vi "GenerateCode.vi"(0 "XRef":T17, 1 "Terms":T14, 2 "Diagram":T13, 3 "State In":T1) -> (14 "Generated Code?":T9, 15 "Reply":T12, 16 "Fatal Error Out":T11, 17 "State Out":T1)   [LabVIEW 2021, in "myRIO AO N Samples Open.xnode"]
uses:
  <vilib>/myRIO/Instrument Drivers/Onboard IO/AO Block/vis/myRIO AO N Samples Open.xnode
  <vilib>/XNodeSupport/XNodeXNodeRef.ctl
  <vilib>/XNodeSupport/XNodeTermIDPairs.ctl
  <vilib>/XNodeSupport/XNodeTermIDPair.ctl
  <vilib>/XNodeSupport/XNodeTermRef.ctl
  <vilib>/XNodeSupport/XNodeString.ctl
  <vilib>/XNodeSupport/XNodeTopLevelDiagramRef.ctl
  <vilib>/myRIO/Instrument Drivers/Onboard IO/AO Block/vis/State.ctl
  <vilib>/myRIO/Common/Instrument Driver Framework/Utilities/typedefs/myRIOXPeripheral.ctl
  <vilib>/XNodeSupport/XNodeTerm4Array.ctl
  <vilib>/XNodeSupport/XNodeTerm4.ctl
  <vilib>/XNodeSupport/XNodeVariant.ctl
  <vilib>/XNodeSupport/XNodeRect32.ctl
  <vilib>/XNodeSupport/XNodeInt.ctl
  <vilib>/XNodeSupport/XNodeBool.ctl
  <vilib>/XNodeSupport/XNodeTermDirection.ctl
  <vilib>/XNodeSupport/XNodeStringArray.ctl
  <vilib>/XNodeSupport/XNodeErrorCluster.ctl
  <vilib>/userdefined/High Color/nirio_resource_hc.ctl
  <vilib>/XNodeSupport/NI_XNodeSupport.lvlib
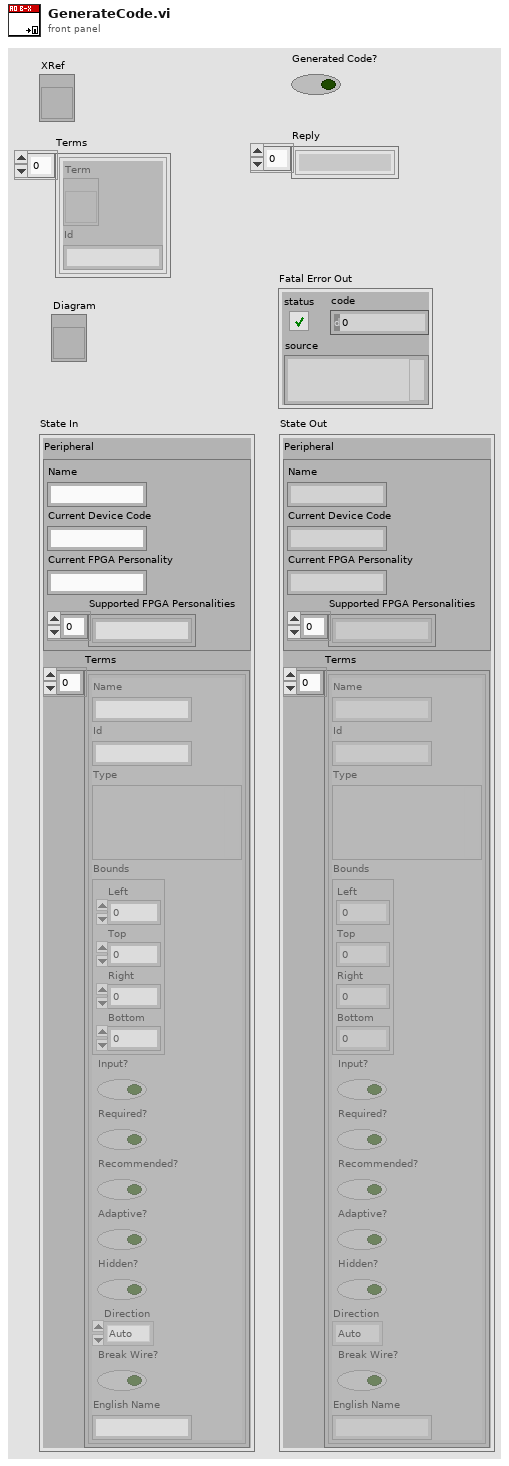
[diagram p1: front panel]
types:
  T1 = typedef "myRIO AO N Samples Open.xnode/State.ctl" = cluster{"Peripheral":T2, "Terms":T3}
  T2 = typedef "myRIOXPeripheral.ctl" = cluster{"Name":string, "Current Device Code":string, "Current FPGA Personality":string, "Supported FPGA Personalities":string[]}
  T3 = typedef "NI_XNodeSupport.lvlib/XNodeTerm4Array.ctl" = T4[]
  T4 = typedef "NI_XNodeSupport.lvlib/XNodeTerm4.ctl" = cluster{"Name":T5, "Id":T5, "Type":T6, "Bounds":T7, "Input?":T9, "Required?":T9, "Recommended?":T9, "Adaptive?":T9, "Hidden?":T9, "Direction":T10, "Break Wire?":T9, "English Name":T5}
  T5 = typedef "NI_XNodeSupport.lvlib/XNodeString.ctl" = string
  T6 = typedef "NI_XNodeSupport.lvlib/XNodeVariant.ctl" = variant
  T7 = typedef "NI_XNodeSupport.lvlib/XNodeRect32.ctl" = cluster{"Left":T8, "Top":T8, "Right":T8, "Bottom":T8}
  T8 = typedef "NI_XNodeSupport.lvlib/XNodeInt.ctl" = i32
  T9 = typedef "NI_XNodeSupport.lvlib/XNodeBool.ctl" = bool
  T10 = typedef "NI_XNodeSupport.lvlib/XNodeTermDirection.ctl" = enum32{"Auto", "Up", "Down", "Left", "Right", "Center"}
  T11 = typedef "NI_XNodeSupport.lvlib/XNodeErrorCluster.ctl" = errorcluster
  T12 = typedef "NI_XNodeSupport.lvlib/XNodeStringArray.ctl" = T5[]
  T13 = typedef "NI_XNodeSupport.lvlib/XNodeTopLevelDiagramRef.ctl" = refnum<vi>
  T14 = typedef "NI_XNodeSupport.lvlib/XNodeTermIDPairs.ctl" = T15[]
  T15 = typedef "NI_XNodeSupport.lvlib/XNodeTermIDPair.ctl" = cluster{"Term":T16, "Id":T5}
  T16 = typedef "NI_XNodeSupport.lvlib/XNodeTermRef.ctl" = refnum<vi>
  T17 = typedef "NI_XNodeSupport.lvlib/XNodeXNodeRef.ctl" = refnum<vi>
  T18 = typedef "nirio_resource_hc.ctl" = tag
  T19 = typedef "LVPositionTypeDef.ctl" = cluster{"Left":i32, "Top":i32}
  T20 = typedef "Hardware Version Enum.ctl" = enum16{"Unknown", "myRIO-1900", "myRIO-1950", "roboRIO", "NI ELVIS RIO CM", "ELVIS III"}
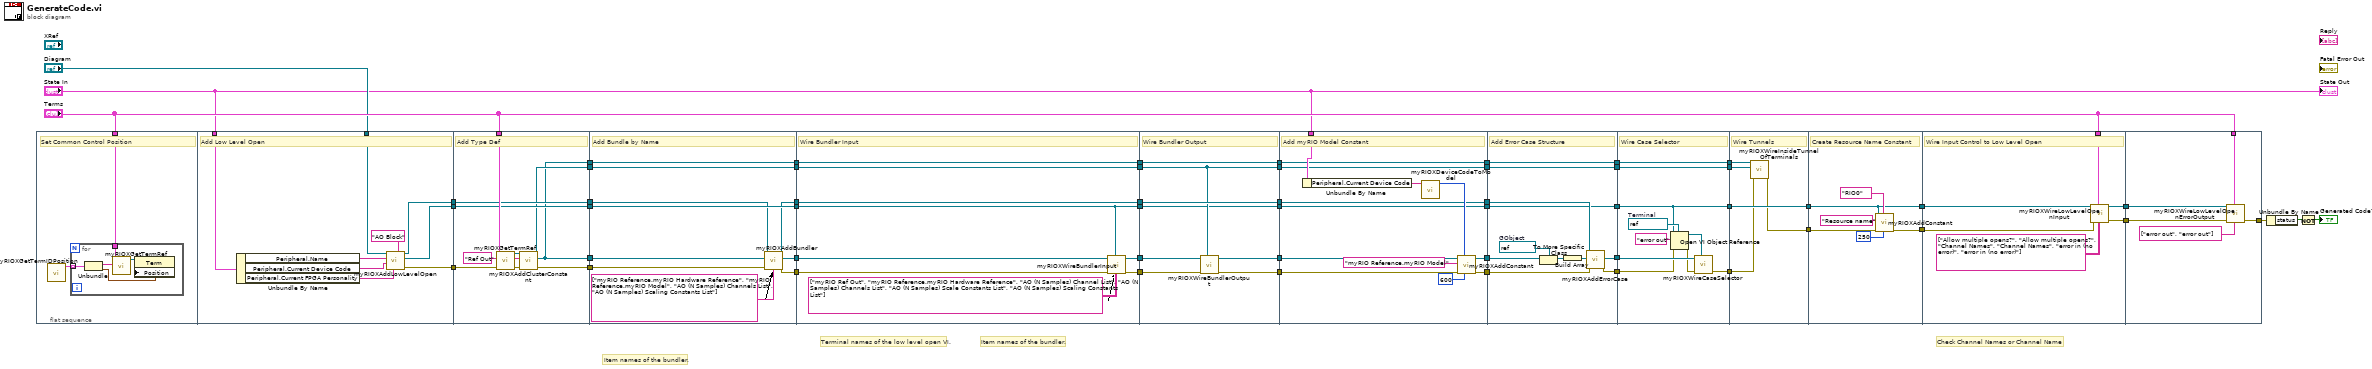
[diagram p0: block diagram]
diagram:
  # "Check Channel Names or Channel Name"
  # "Item names of the bundler."
  # "Terminal names of the low level open VI."
  # "Item names of the bundler."
  n1 = flat-sequence {
    tunnel: "Terms" -> [w56]
    tunnel: "State In" -> [w70]
    tunnel: "Diagram" -> [w69]
    tunnel: [w67] -> w53
    tunnel: [w68] -> w52
    tunnel: [w66] -> w51
    tunnel: "Terms" -> [w80]
    tunnel: [w76] -> w50
    tunnel: [w79] -> w49
    tunnel: w53 -> [w79]
    tunnel: [w78] -> w48
    tunnel: w52 -> [w78]
    tunnel: [w77] -> w47
    tunnel: [w76] -> w46
    tunnel: [w75] -> w45
    tunnel: w51 -> [w74]
    tunnel: w50 -> [w90]
    tunnel: w49 -> [w87]
    tunnel: [w89] -> w44
    tunnel: [w88] -> w43
    tunnel: w48 -> [w88]
    tunnel: [w86] -> w42
    tunnel: w47 -> [w85]
    tunnel: [w85] -> w41
    tunnel: [w84] -> w40
    tunnel: w46 -> [w84]
    tunnel: w45 -> [w83]
    tunnel: [w82] -> w39
    tunnel: w44 -> [w99]
    tunnel: w43 -> [w94]
    tunnel: [w98] -> w38
    tunnel: [w97] -> w37
    tunnel: w42 -> [w97]
    tunnel: [w96] -> w36
    tunnel: w41 -> [w96]
    tunnel: [w95] -> w35
    tunnel: w40 -> [w95]
    tunnel: [w94] -> w34
    tunnel: w39 -> [w93]
    tunnel: [w92] -> w33
    tunnel: w38 -> [w107]
    tunnel: [w104] -> w32
    tunnel: w37 -> [w106]
    tunnel: [w106] -> w31
    tunnel: w36 -> [w103]
    tunnel: [w103] -> w30
    tunnel: w35 -> [w105]
    tunnel: [w105] -> w29
    tunnel: [w102] -> w28
    tunnel: w34 -> [w102]
    tunnel: w33 -> [w101]
    tunnel: [w100] -> w27
    tunnel: w32 -> [w120]
    tunnel: "State In" -> [w118]
    tunnel: [w114] -> w26
    tunnel: w31 -> [w114]
    tunnel: [w113] -> w25
    tunnel: [w112] -> w24
    tunnel: w30 -> [w112]
    tunnel: [w111] -> w23
    tunnel: w29 -> [w111]
    tunnel: w28 -> [w110]
    tunnel: [w110] -> w22
    tunnel: w27 -> [w109]
    tunnel: [w108] -> w21
    tunnel: w26 -> [w131]
    tunnel: w25 -> [w130]
    tunnel: [w126] -> w20
    tunnel: w24 -> [w126]
    tunnel: [w125] -> w19
    tunnel: w23 -> [w125]
    tunnel: [w124] -> w18
    tunnel: w22 -> [w124]
    tunnel: [w123] -> w17
    tunnel: w21 -> [w122]
    tunnel: [w121] -> w16
    tunnel: w20 -> [w141]
    tunnel: [w141] -> w15
    tunnel: w19 -> [w140]
    tunnel: [w140] -> w14
    tunnel: w18 -> [w136]
    tunnel: [w136] -> w13
    tunnel: w17 -> [w139]
    tunnel: w16 -> [w132]
    tunnel: [w134] -> w12
    tunnel: w15 -> [w145]
    tunnel: w14 -> [w146]
    tunnel: [w144] -> w11
    tunnel: w13 -> [w144]
    tunnel: w12 -> [w143]
    tunnel: [w142] -> w10
    tunnel: w11 -> [w149]
    tunnel: [w149] -> w9
    tunnel: w10 -> [w148]
    tunnel: [w147] -> w8
    tunnel: w9 -> [w157]
    tunnel: "Terms" -> [w158]
    tunnel: [w156] -> w7
    tunnel: [w155] -> w6
    tunnel: w8 -> [w154]
    tunnel: [w162] -> w5
    tunnel: w7 -> [w163]
    tunnel: w6 -> [w161]
    tunnel: "Terms" -> [w160]
    frame #0 {
      # "Set Common Control Position"
      n2 = call <vilib>:"myRIOXGetTermIDPosition.vi"() -> ("Term ID Postion"=w55:cluster{"Term ID":string, "Position":T19}[])  [unwired: 11 in]
      n3 = for {
        tunnel: w56 -> [w61]
        tunnel: w55 -> [w59] mode=indexing
        n4 = Unbundle(w59) -> ("Term ID"=w58:string, "Position"=w57:T19)
        n5 = call <vilib>:"myRIOXGetTermRef.vi"("Term ID"=w58, "Terms"=w61) -> ("Terminal Reference"=w60:T16)  [unwired: 7 in, 2 out]
        n6 = property class="Term"(reference=w60, "Position"=w57) -> ()  [unwired: 1 in, 2 out]
      }
    }
    frame #1 {
      # "Add Low Level Open"
      n7 = Unbundle By Name(w70) -> ("Peripheral.Name"=w63:string, "Peripheral.Current Device Code"=w65:string, "Peripheral.Current FPGA Personality"=w64:string)
      n8 = call <vilib>:"myRIOXAddLowLevelOpen.vi"("Peripheral Name"="AO Block", "FPGA Personality"=w64, "Device Code"=w65, "VI Name"=w63, "Diagram Reference"=w69) -> ("error out"=w66:errorcluster, "SubVI Reference"=w68:refnum<vi>, "Duplicated Diagram Reference"=w67:T13)  [unwired: 4 in]
    }
    frame #2 {
      # "Add Type Def"
      n9 = call <vilib>:"myRIOXGetTermRef.vi"("Term ID"="Ref Out", "Terms"=w80) -> ("Full Term ID"=w72:T5, "Terminal Reference"=w71:T16)  [unwired: 7 in, 1 out]
      n10 = call <vilib>:"myRIOXAddClusterConstant.vi"("error in (no error)"=w74, "Full Term ID"=w72, "Term Reference"=w71) -> ("error out"=w75:errorcluster, "Cluster Constant Terminal Reference"=w76:refnum<vi>, "Duplicated Term Reference"=w77:T16)  [unwired: 6 in]
    }
    frame #3 {
      # "Add Bundle by Name"
      n11 = call <vilib>:"myRIOXAddBundler.vi"("Element Names"=string[] ["myRIO Reference.myRIO Hardware Reference", "myRIO Reference.myRIO Model", "AO (N Samples) Channels List", "AO (N Samples) Scaling Constants List"], "error in (no error)"=w83, "Cluster Constant Terminal Reference"=w90, "Diagram Reference"=w87) -> ("error out"=w82:errorcluster, "Named Bundler Reference"=w89:refnum<vi>, "Duplicated Diagram Reference"=w86:T13)  [unwired: 5 in]
    }
    frame #4 {
      # "Wire Bundler Input"
      n12 = call <vilib>:"myRIOXWireBundlerInput.vi"("Wiring Specs"=string[][] [["myRIO Ref Out", "myRIO Reference.myRIO Hardware Reference"], ["AO (N Samples) Channel List", "AO (N Samples) Channels List"], ["AO (N Samples) Scale Constants List", "AO (N Samples) Scaling Constants List"]], "SubVI Reference"=w94, "error in (no error)"=w93, "Named Bundler Reference"=w99) -> ("error out"=w92:errorcluster, "Duplicated Named Bundler Reference"=w98:refnum<vi>)  [unwired: 6 in]
    }
    frame #5 {
      # "Wire Bundler Output"
      n13 = call <vilib>:"myRIOXWireBundlerOutput.vi"("Sink Terminam Reference"=w103, "error in (no error)"=w101, "Named Bundler Reference"=w107) -> ("error out"=w100:errorcluster, "Duplicated Named Bundler Reference"=w104:refnum<vi>)  [unwired: 7 in]
    }
    frame #6 {
      # "Add myRIO Model Constant"
      n14 = Unbundle By Name(w118) -> ("Peripheral.Current Device Code"=w117:string)
      n15 = call <vilib>:"myRIOXDeviceCodeToModel.vi"("Device Code"=w117) -> ("myRIO Reference.myRIO Model"=w116:T20)  [unwired: 10 in]
      n16 = call <vilib>:"myRIOXAddConstant.vi"("Left (0)"=600 ("Left"), "Value"=w116, "error in (no error)"=w109, "Terminal Name"="myRIO Reference.myRIO Model", "Owner Reference"=w120) -> ("error out"=w108:errorcluster, "Duplicated Owner Reference"=w113:refnum<vi>)  [unwired: 5 in]
    }
    frame #7 {
      w127 = refnum<vi> refnum  # GObject
      # "Add Error Case Structure"
      n17 = To More Specific Class(target class=w127, reference=w130) -> (specific class reference=w128:refnum<vi>)  [unwired: 1 in, 1 out]
      n18 = Build Array(w128) -> (w129:refnum<vi>[])
      n19 = call <vilib>:"myRIOXAddErrorCase.vi"("error in (no error)"=w122, "Enclosed Object References"=w129, "Diagram Reference"=w131) -> ("error out"=w121:errorcluster, "Case Structure Reference"=w123:refnum<vi>)  [unwired: 6 in, 1 out]
    }
    frame #8 {
      w138 = refnum<vi> refnum  # Terminal
      # "Wire Case Selector"
      n20 = Open VI Object Reference(7:w138, 8:w132, 10:"error out" ("name/order"), 11:w136) -> (0:w133:errorcluster, 3:w137:refnum<vi>)
      n21 = call <vilib>:"myRIOXWireCaseSelector.vi"("Source Terminam Reference"=w137, "error in (no error)"=w133, "Case Structure Reference"=w139) -> ("error out"=w134:errorcluster)  [unwired: 7 in, 1 out]
    }
    frame #9 {
      # "Wire Tunnels"
      n22 = call <vilib>:"myRIOXWireInsideTunnelOfTerminals.vi"("error in (no error)"=w143, "Sink Terminam Reference"=w145, "Source Terminam Reference"=w146) -> ("error out"=w142:errorcluster)  [unwired: 6 in, 2 out]
    }
    frame #10 {
      # "Create Resource Name Constant"
      n23 = call <vilib>:"myRIOXAddConstant.vi"("Left (0)"=250 ("Left"), "Value"=T18 "RIO0" ("Resource name"), "error in (no error)"=w148, "Terminal Name"="Resource name", "Owner Reference"=w149) -> ("error out"=w147:errorcluster)  [unwired: 5 in, 1 out]
    }
    frame #11 {
      # "Wire Input Control to Low Level Open"
      n24 = call <vilib>:"myRIOXWireLowLevelOpenInput.vi"("Wiring Specs"=string[][] [["Allow multiple opens?", "Allow multiple opens?"], ["Channel Names", "Channel Names"], ["error in (no error)", "error in (no error)"]], "Terms"=w158, "error in (no error)"=w154, "SubVI Reference"=w157) -> ("error out"=w156:errorcluster, "Duplicated SubVI Reference"=w155:refnum<vi>)  [unwired: 6 in]
    }
    frame #12 {
      n25 = call <vilib>:"myRIOXWireLowLevelOpenErrorOutput.vi"("Wiring Specs"=string[] ["error out", "error out"], "Terms"=w160, "error in (no error)"=w163, "SubVI Reference"=w161) -> ("error out"=w162:errorcluster)  [unwired: 6 in, 1 out]
    }
  }
  n26 = Unbundle By Name(w5) -> ("status"=w4:bool)
  n27 = Not(x=w4) -> (.not. x?=→"Generated Code?":bool)
  "State Out" <- "State In"
